vi "1 step.vi"(5 "PH1":dbl, 6 "УЗ2":dbl, 7 "УЗ1":dbl) -> (0 "Error output":bool=TRUE, 1 "ДН1 объем подачи":dbl format="%#_13g", 2 "Дозирующий насос 1":bool=TRUE, 3 "Насос 1":bool=TRUE)   [LabVIEW 2019]
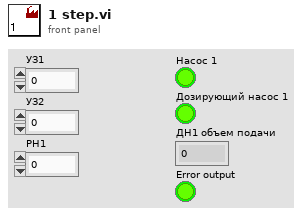
[diagram p1: front panel]
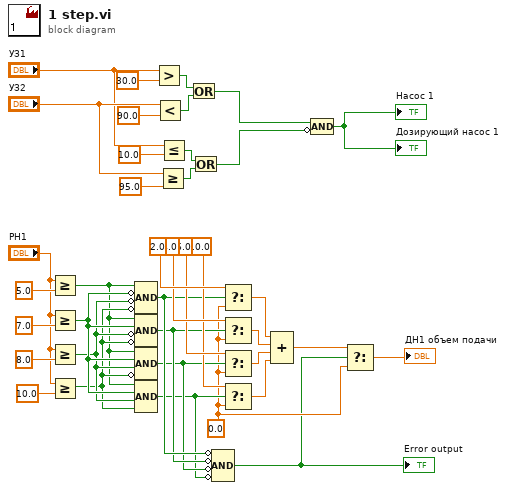
[diagram p0: block diagram]
diagram:
  w2 = 0.0
  n1 = Greater Or Equal?(x="PH1", y=5.0) -> (x >= y?=w28:bool)
  n2 = Greater Or Equal?(x="PH1", y=7.0) -> (x >= y?=w31:bool)
  n3 = Greater Or Equal?(x="PH1", y=8.0) -> (x >= y?=w30:bool)
  n4 = Greater Or Equal?(x="PH1", y=10.0) -> (x >= y?=w29:bool)
  n5 = Compound Arithmetic op=AND(w28, invert w31, invert w30, invert w29) -> (w8:bool)
  n6 = Compound Arithmetic op=AND(w28, w31, invert w30, invert w29) -> (w7:bool)
  n7 = Compound Arithmetic op=AND(w28, w31, w30, invert w29) -> (w6:bool)
  n8 = Compound Arithmetic op=AND(w28, w31, w30, w29) -> (w5:bool)
  n9 = Greater?(x="УЗ1", y=30.0) -> (0:w19:bool)
  n10 = Less?(x="УЗ2", y=90.0) -> (x < y?=w18:bool)
  n11 = Greater Or Equal?(x="УЗ2", y=95.0) -> (x >= y?=w12:bool)
  n12 = Less Or Equal?(x="УЗ1", y=10.0) -> (x <= y?=w13:bool)
  n13 = Or(x=w19, y=w18) -> (x .or. y?=w10:bool)
  n14 = Or(x=w13, y=w12) -> (x .or. y?=w11:bool)
  n15 = Compound Arithmetic op=AND(invert w8, invert w7, invert w6, invert w5) -> (w1:bool)
  "Error output" <- w1
  n16 = Select(t=2.0, s=w8, f=w2) -> (s? t:f=w23:dbl)
  n17 = Select(t=4.0, s=w7, f=w2) -> (s? t:f=w22:dbl)
  n18 = Select(t=6.0, s=w6, f=w2) -> (s? t:f=w21:dbl)
  n19 = Select(t=10.0, s=w5, f=w2) -> (s? t:f=w20:dbl)
  n20 = Compound Arithmetic op=ADD(w23, w22, w21, w20) -> (w4:dbl)
  n21 = Compound Arithmetic op=AND(w10, invert w11) -> (→"Насос 1" →"Дозирующий насос 1":bool)
  n22 = Select(t=w4, s=w1, f=w2) -> (s? t:f=→"ДН1 объем подачи":dbl)
